vi "Get Light Stack Prepend.vi"(8 "error in":errorcluster, 11 "MiniIO in":refnum<class "MiniIO.lvclass">) -> (0 "error out":errorcluster, 1 "Blink Memory":bool[](array[boolean]), 2 "D/O Prepend":bool[](array[boolean]), 3 "MiniIO out":refnum<class "MiniIO.lvclass">)   [LabVIEW 2018, in "MiniIO.lvlib" / "MiniIO.lvclass"]
uses:
  MiniIO.lvclass
  PPLs/PLC/Light Stack/Light Stack.lvlibp/Light Stack.lvclass
  PPLs/PLC/Parent/PLC.lvlibp/PLC.lvclass
  C:/AME Test Engineering/LabVIEW/PPLs/PLC/Parent/PLC.lvlibp/PLC.lvclass
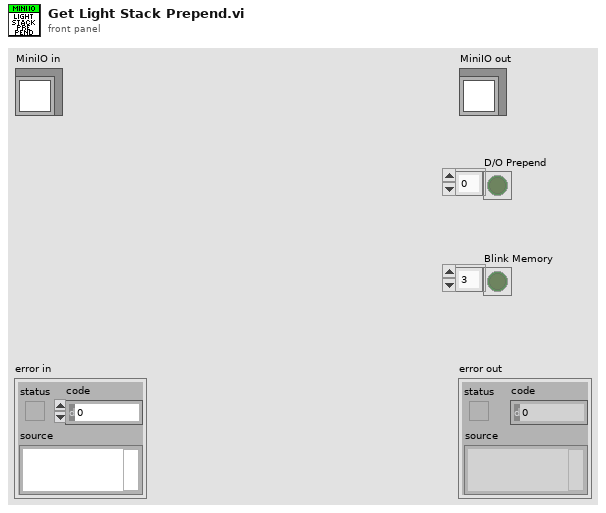
[diagram p1: front panel]
types:
  T1 = typedef "Light Stack.lvlibp/Light Mode.ctl" = enum16{"OFF", "ON", "BLINK"}
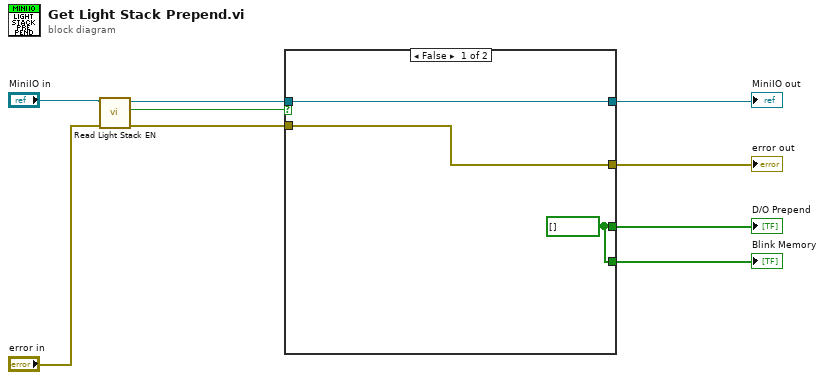
[diagram p0: block diagram]
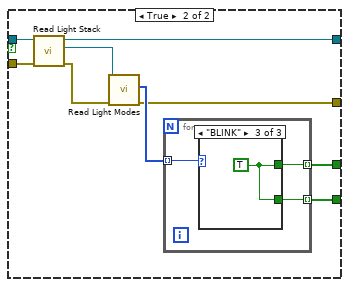
[diagram p2: hidden frame]
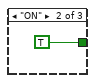
[diagram p4: hidden frame]
diagram:
  n1 = call "Read Light Stack EN.vi"("error in (no error)"="error in", "PLC in"="MiniIO in") -> ("error out"=w2:errorcluster, "Light Stack?"=w4:bool, "PLC out"=w3:refnum<class "MiniIO.lvclass">)  [unwired: 7 in]
  n2 = case shown="False" w4 {
    tunnel: w2 -> [w12 w16]
    tunnel: [w12 w20] -> w9
    tunnel: [w11 w19] -> w8
    tunnel: [w11 w18] -> w7
    tunnel: w3 -> [w10 w17]
    tunnel: [w10 w13] -> w1
    frame False {
      w11 = bool[] []
    }
    frame True {
      n3 = call "Read Light Stack.vi"("error in (no error)"=w16, "PLC in"=w17) -> ("error out"=w14:errorcluster, "Light Stack"=w15:refnum<class "Light Stack.lvclass">, "PLC out"=w13:refnum<class "MiniIO.lvclass">)  [unwired: 7 in]
      n4 = call "Read Light Modes.vi"("error in (no error)"=w14, "Light Stack in"=w15) -> ("error out"=w20:errorcluster, "Light Modes"=w21:T1[])  [unwired: 7 in, 1 out]
      n5 = for {
        tunnel: w21 -> [w24] mode=indexing
        tunnel: [w23] -> w19 mode=indexing
        tunnel: [w22] -> w18 mode=indexing
        n6 = case shown="\"BLINK\"" w24 {
          tunnel: [_ TRUE w26] -> w23
          tunnel: [_ _ w26] -> w22
          frame "OFF", Default {
          }
          frame "ON" {
          }
          frame "BLINK" {
            w26 = TRUE
          }
        }
      }
    }
  }
  "error out" <- w9
  "MiniIO out" <- w1
  "D/O Prepend" <- w8
  "Blink Memory" <- w7
